vi "Example_ConsoleWriter.vi"() -> ()   [LabVIEW 2024, in "ConsoleWriter.lvclass"]
uses:
  ConsoleWriter.lvclass
  ConsoleWriter.lvclass/ConsoleWriter.ctl
panel:
  out "error out":errorcluster
  in  "stop":bool
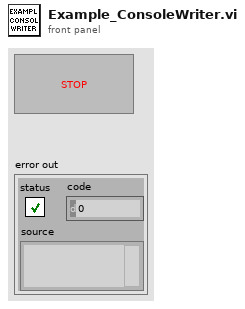
[diagram p1: front panel]
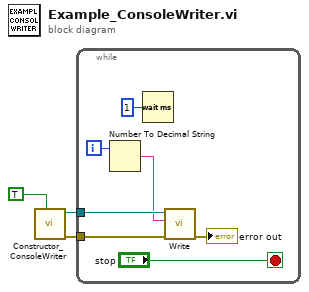
[diagram p0: block diagram]
diagram:
  n1 = call "Constructor_ConsoleWriter.vi"("Autoshow? (f)"=TRUE) -> ("error out"=w2:errorcluster, "ConsoleWriter out"=w1:refnum<class "ConsoleWriter.lvclass">)  [unwired: 9 in]
  n2 = while {
    tunnel: w2 -> [w9]
    tunnel: w1 -> [w8]
    i -> [w5]
    stop <- "stop" stop-if-true
    n3 = Number To Decimal String(number=w5) -> (decimal integer string=w4:string)  [unwired: 1 in]
    n4 = Wait (ms)(milliseconds to wait=u32 1) -> ()  [unwired: 1 out]
    n5 = call-dynamic "Write.vi"("error in (no error)"=w9, "Message"=w4, "ConsoleWriter in"=w8) -> ("error out"=→"error out":errorcluster)  [unwired: 7 in, 1 out]
  }
